vi "excel读取.vi"(6 "选取数据列":i32, 9 "路径":path, 10 "Excel._Application":refnum<k7>, 11 "自动化引用句柄输入":refnum<k7>) -> (2 "数组":string[](array[string]), 3 "表格":string[][](table))   [LabVIEW 2016]
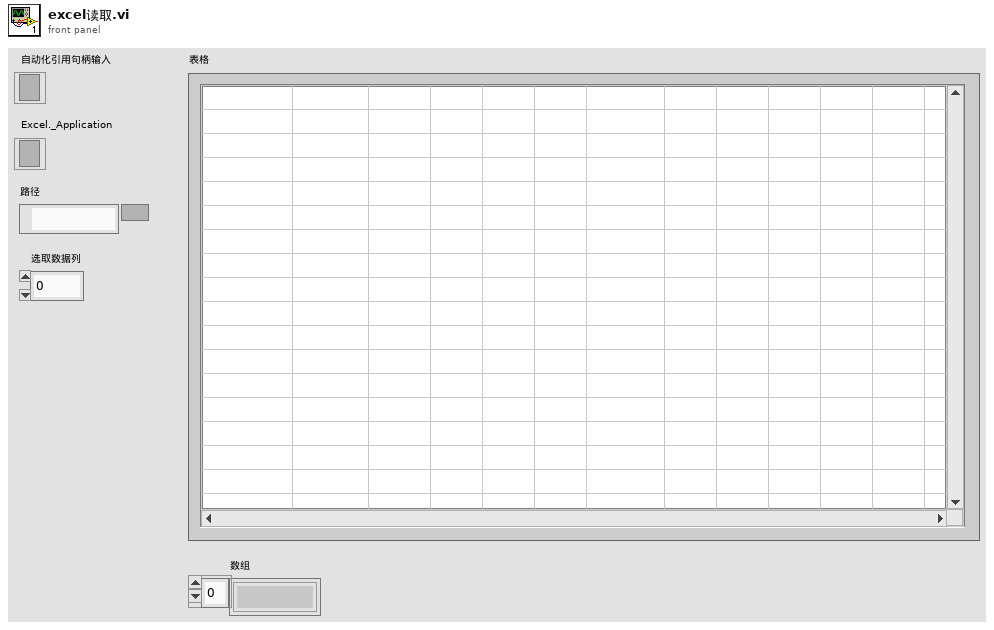
[diagram p1: front panel]
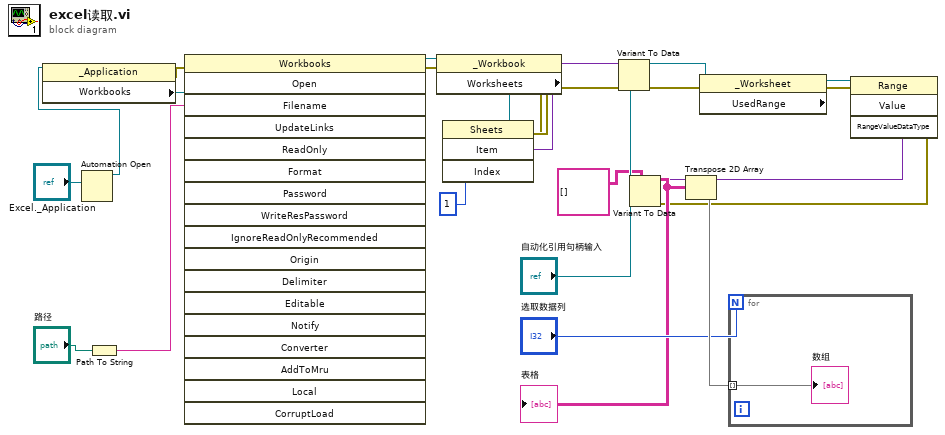
[diagram p0: block diagram]
diagram:
  n1 = Automation Open(Automation Refnum="Excel._Application") -> (Automation Refnum=w21:refnum<k7>)  [unwired: 3 in, 1 out]
  n2 = property class="_Application"(reference=w21) -> (error out=w19:errorcluster, "Workbooks"=w20:refnum<k7>)  [unwired: 1 in, 1 out]
  n3 = Path To String ("路径至字符串转换")(path="路径") -> (string=w17:string)
  n4 = invoke class="Workbooks" method="Open"(reference=w20, error in=w19, "Filename"=w17) -> (error out=w15:errorcluster, "Open"=w16:refnum<k7>)  [unwired: 15 in, 16 out]
  n5 = property class="_Workbook"(reference=w16, error in=w15) -> (error out=w12:errorcluster, "Worksheets"=w13:refnum<k7>)  [unwired: 1 out]
  n6 = invoke class="Sheets" method="Item"(reference=w13, error in=w12, "Index"=1) -> (error out=w10:errorcluster, "Item"=w11:variant)  [unwired: 1 in, 2 out]
  n7 = Variant To Data(error in=w10, type="自动化引用句柄输入", Variant=w11) -> (data=w8:refnum<k7>, error out=w7:errorcluster)
  n8 = property class="_Worksheet"(reference=w8, error in=w7) -> (error out=w5:errorcluster, "UsedRange"=w6:refnum<k7>)  [unwired: 1 out]
  n9 = invoke class="Range" method="Value"(reference=w6, error in=w5) -> (error out=w3:errorcluster, "Value"=w4:variant)  [unwired: 2 in, 2 out]
  n10 = Variant To Data(error in=w3, type=string[][] [], Variant=w4) -> (data=w22:string[][])  [unwired: 1 out]
  "表格" <- w22
  n11 = Transpose 2D Array(2D array=w22) -> (transposed array=w24:string[][])
  n12 = for {
    N: "选取数据列" -> [_]
    tunnel: w24 -> [w25] mode=indexing
    "数组" <- w25
  }
